vi "CollectSensorData.vi"(0 "Serial buffer":string) -> (2 "Grip Force":dbl, 3 "Static Futek Volts":dbl, 4 "Dynamic Load Force":dbl)   [LabVIEW 2020]
doc: "VI for GF and LF conversion."
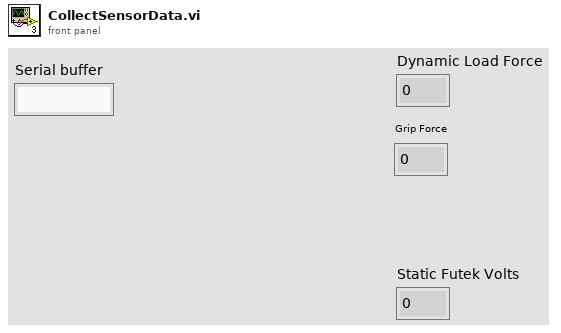
[diagram p1: front panel]
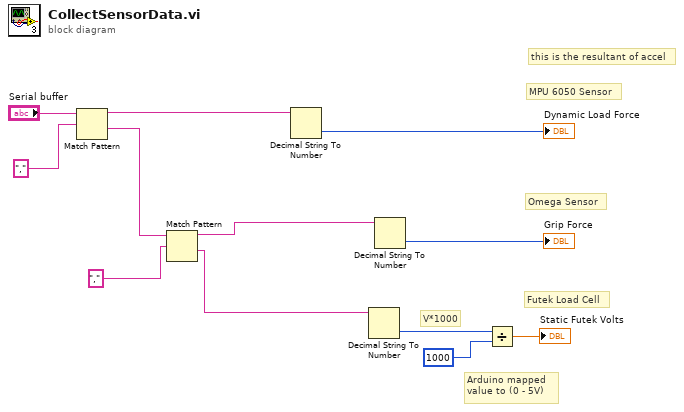
[diagram p0: block diagram]
diagram:
  # "this is the resultant of accel"
  # "V*1000"
  # "Omega Sensor"
  # "Futek Load Cell"
  # "MPU 6050 Sensor"
  # "Arduino mapped\nvalue to (0 - 5V)"
  n1 = Match Pattern(string="Serial buffer", regular expression=",") -> (before substring=w12:string, after substring=w10:string)  [unwired: 1 in, 2 out]
  n2 = Match Pattern(string=w10, regular expression=",") -> (before substring=w9:string, after substring=w1:string)  [unwired: 1 in, 2 out]
  n3 = Decimal String To Number(string=w12) -> (number=→"Dynamic Load Force":i32)  [unwired: 2 in, 1 out]
  n4 = Decimal String To Number(string=w1) -> (number=w6:i32)  [unwired: 2 in, 1 out]
  n5 = Decimal String To Number(string=w9) -> (number=→"Grip Force":i32)  [unwired: 2 in, 1 out]
  n6 = Divide(x=w6, y=1000) -> (x/y=→"Static Futek Volts":dbl)
